vi "image_save.vi"() -> ()   [LabVIEW 2011]
panel:
  in  "File Path":path
  in  "error in":errorcluster
  out "Image Out":T1(plugin-control)
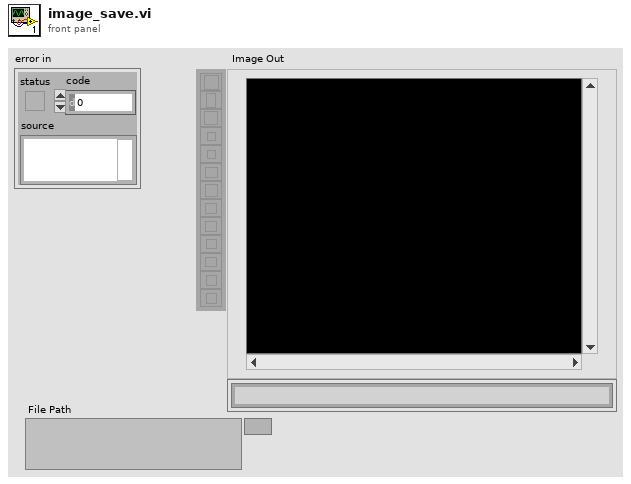
[diagram p1: front panel]
types:
  T1 = typedef "IMAQ Image.ctl" = refnum<image>
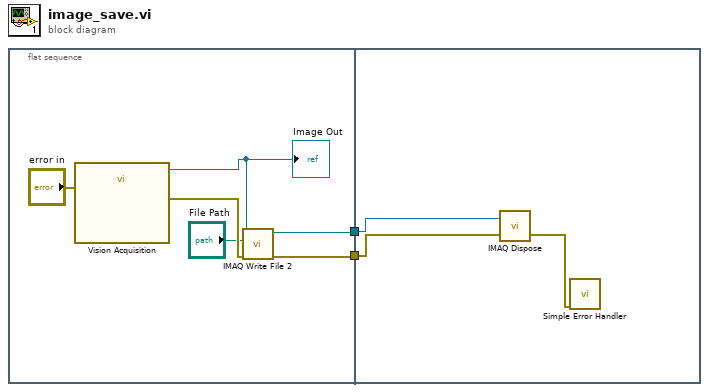
[diagram p0: block diagram]
diagram:
  n1 = flat-sequence {
    tunnel: [w5] -> w2
    tunnel: [w4] -> w1
    tunnel: w2 -> [w11]
    tunnel: w1 -> [w10]
    frame #0 {
      n2 = call "Vision Acquisition"("error in"="error in") -> ("Image Out"=w6:T1, "error out"=w7:errorcluster)  [unwired: 25 in]
      "Image Out" <- w6
      n3 = call-poly "IMAQ Write File 2"("error in (no error)"=w7, "File Path"="File Path", "Image"=w6) -> ("error out"=w4:errorcluster, "Image Out (duplicate)"=w5:T1)  [unwired: 7 in]
    }
    frame #1 {
      n4 = call "IMAQ Dispose"("Image"=w11, "error in (no error)"=w10) -> ("error out"=w9:errorcluster)  [unwired: 4 in]
      n5 = call <vilib>:"Simple Error Handler.vi"("error in (no error)"=w9) -> ()  [unwired: 4 in, 5 out]
    }
  }
